vi "swerve_open_module.vi"(0 "Module Suffix":string, 5 "Drive CAN ID":u8, 7 "Azimuth CAN ID":u8, 9 "Encoder CAN ID":u8, 11 "error in":errorcluster, 12 "Encoder Offset (Deg)":dbl) -> (15 "error out":errorcluster)   [LabVIEW 2020]
uses:
  <vilib>/Rock Robotics/WPI/ThirdParty/Phoenix-LabVIEW/CANCoder/Controls/CTRE_Phoenix_CANcoder_AbsoluteSensorRange.ctl
  <vilib>/Rock Robotics/WPI/ThirdParty/Phoenix-LabVIEW/CANCoder/Controls/CTRE_Phoenix_CANcoder_StatusFrame.ctl
  <vilib>/Rock Robotics/WPI/ThirdParty/Phoenix-LabVIEW/Motor Controller/Controls/CTRE_Phoenix_MotorControl_FeedbackDevice_TalonFX.ctl
  <vilib>/Rock Robotics/WPI/ThirdParty/Phoenix-LabVIEW/Motor Controller/Controls/CTRE_Phoenix_MotorControl_RemoteSourceType.ctl
  <vilib>/Rock Robotics/WPI/ThirdParty/Phoenix-LabVIEW/Motor Controller/Controls/CTRE_Phoenix_MotorControl_NeutralMode.ctl
  <vilib>/Rock Robotics/WPI/ThirdParty/Phoenix-LabVIEW/CANCoder/Controls/CTRE_Phoenix_CANcoder_SensorInitializationStrategy.ctl
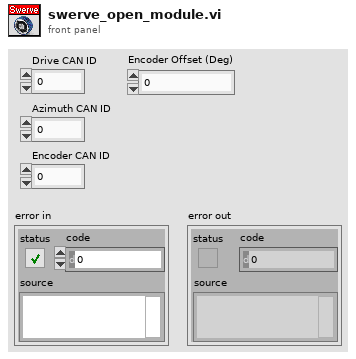
[diagram p1: front panel]
types:
  T1 = typedef "CTRE_Phoenix_CANcoder_StatusFrame.ctl" = u32
  T2 = typedef "CTRE_Phoenix_CANcoder_AbsoluteSensorRange.ctl" = enum16{"Unsigned [0 to 360)", "Signed [-180 to +180)"}
  T3 = typedef "CTRE_Phoenix_MotorControl_NeutralMode.ctl" = enum8{"EEPROMSetting", "Override to Coast", "Override to Brake"}
  T4 = typedef "CTRE_Phoenix_MotorControl_FeedbackDevice_TalonFX.ctl" = i8
  T5 = typedef "CTRE_Phoenix_MotorControl_RemoteSourceType.ctl" = enum16{"Off", "Talon SRX Selected Sensor", "Pigeon IMU Yaw", "Pigeon IMU Pitch", "Pigeon IMU Roll", "CANifier Quadrature", "CANifier PWM Input 0", "CANifier PWM Input 1", "CANifier PWM Input 2", "CANifier PWM Input 3", "Gadgeteer Pigeon Yaw", "Gadgeteer Pigeon Pitch", "Gadgeteer Pigeon Roll", "CANCoder"}
  T6 = typedef "CTRE_Phoenix_CANcoder_SensorInitializationStrategy.ctl" = enum16{"Boot To Zero", "Boot To Absolute Position"}
  T7 = typedef "WPI_MotorControlDeviceRef.ctl" = cluster{"DeviceStatus":errorcluster, "Type":T8, "PWM":cluster{"PWM Channel":T9, "DeadBand":T10}, "CAN":cluster{"Device Number":u8, "SetOutput VI Ref":variant, "GetOutput VI Ref":variant, "Enable VI Ref":variant, "Disable VI Ref":variant, "Data":variant}, "Invert":bool, "DIO PWM":cluster{"PWM \"Enable\" Channel":T9, "DIOChannel":T11, "PWM Rate":dbl}}
  T8 = typedef "WPI_MotorControlType.ctl" = enum16{"PWM", "CAN", "DIO PWM"}
  T9 = typedef "FPGA_DIOPWMChannel.ctl" = enum8{"PWM 0", "PWM 1", "PWM 2", "PWM 3", "PWM 4", "PWM 5", "PWM 6", "PWM 7", "PWM 8", "PWM 9", "PWM MXP 0", "PWM MXP 1", "PWM MXP 2", "PWM MXP 3", "PWM MXP 4", "PWM MXP 5", "PWM MXP 6", "PWM MXP 7", "PWM MXP 8", "PWM MXP 9", "Invalid"}
  T10 = typedef "WPI_PWMDeadband.ctl" = cluster{"Name":string, "maxPositivePwm":i32, "minPositivePwm":i32, "centerPwm":i32, "maxNegativePwm":i32, "minNegativePwm":i32, "angularRange":u16}
  T11 = typedef "FPGA_DIOChannel.ctl" = enum8{"DIO 0", "DIO 1", "DIO 2", "DIO 3", "DIO 4", "DIO 5", "DIO 6", "DIO 7", "DIO 8", "DIO 9", "DIO MXP 0", "DIO MXP 1", "DIO MXP 2", "DIO MXP 3", "DIO MXP 4", "DIO MXP 5", "DIO MXP 6", "DIO MXP 7", "DIO MXP 8", "DIO MXP 9", "DIO MXP 10", "DIO MXP 11", "DIO MXP 12", "DIO MXP 13", "DIO MXP 14", "DIO MXP 15", "SPI Port CS1", "SPI Port CS2", "SPI Port CS3", "SPI Port MISO", "SPI Port MOSI", "Invalid"}
  T12 = typedef "CTRE_Phoenix_CANcoder_DeviceRef.ctl" = cluster{"DeviceStatus":errorcluster, "Device Number":u8, "Handle":u64, "UsageFrame":u32, "Library Path":path}
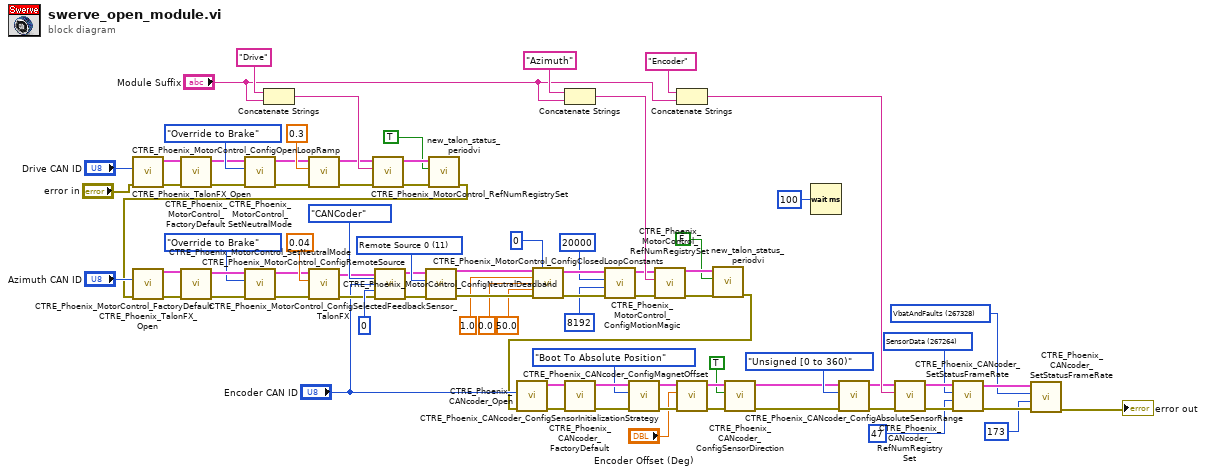
[diagram p0: block diagram]
diagram:
  w11 = T1 267328 items=["SensorData"=267264, "VbatAndFaults"=267328] ("CANcoder Status Frame")
  w21 = T1 267264 items=["SensorData"=267264, "VbatAndFaults"=267328] ("CANcoder Status Frame")
  w59 = T4 11 items=["Integrated Sensor"=1, "Sensor Sum (S0 + S1)"=9, "Sensor Difference (D0 - D1)"=10, "Remote Source 0"=11, "Remote Source 1"=12, "None"=14, "Software Emulated"=15] ("Talon FX Feedback Device")
  n1 = call <vilib>:"CTRE_Phoenix_TalonFX_Open.vi"("error in"="error in", "Device Number"="Drive CAN ID") -> ("error out"=w77:errorcluster, "PhoenixMotorControlDevRef"=w78:T7)  [unwired: 8 in]
  n2 = call <vilib>:"CTRE_Phoenix_MotorControl_FactoryDefault.vi"("error in"=w77, "PhoenixMotorControlDevRef"=w78) -> ("error out"=w30:errorcluster, "PhoenixMotorControlDevRef"=w31:T7)  [unwired: 8 in]
  n3 = call <vilib>:"CTRE_Phoenix_MotorControl_SetNeutralMode.vi"("error in (no error)"=w30, "Motor Control Neutral Mode"=CTRE_Phoenix_MotorControl_NeutralMode."Override to Brake", "PhoenixMotorControlDevRef"=w31) -> ("error out"=w28:errorcluster, "PhoenixMotorControlDevRef"=w29:T7)  [unwired: 7 in]
  n4 = Concatenate Strings("Drive" ("string"), "Module Suffix") -> (w79:string)
  n5 = call <vilib>:"CTRE_Phoenix_MotorControl_ConfigOpenLoopRamp.vi"("error in (no error)"=w28, "secondsFromNeutralToFull"=0.3 ("Drive Ramp (Sec)"), "PhoenixMotorControlDevRef"=w29) -> ("error out"=w26:errorcluster, "PhoenixMotorControlDevRef"=w27:T7)  [unwired: 7 in]
  n6 = call <vilib>:"CTRE_Phoenix_MotorControl_RefNumRegistrySet.vi"("error in (no error)"=w26, "refnum name"=w79, "PhoenixMotorControlDevRef"=w27) -> ("error out"=w4:errorcluster, "PhoenixMotorControlDevRef"=w3:T7)  [unwired: 7 in]
  n7 = call "new_talon_status_periodvi.vi"("error in (no error)"=w4, "Feedback Data?"=TRUE, "PhoenixMotorControlDevRef"=w3) -> ("error out"=w2:errorcluster)  [unwired: 7 in, 1 out]
  n8 = call <vilib>:"CTRE_Phoenix_TalonFX_Open.vi"("error in"=w2, "Device Number"="Azimuth CAN ID") -> ("error out"=w76:errorcluster, "PhoenixMotorControlDevRef"=w75:T7)  [unwired: 8 in]
  n9 = call <vilib>:"CTRE_Phoenix_MotorControl_FactoryDefault.vi"("error in"=w76, "PhoenixMotorControlDevRef"=w75) -> ("error out"=w49:errorcluster, "PhoenixMotorControlDevRef"=w50:T7)  [unwired: 8 in]
  n10 = call <vilib>:"CTRE_Phoenix_MotorControl_SetNeutralMode.vi"("error in (no error)"=w49, "Motor Control Neutral Mode"=CTRE_Phoenix_MotorControl_NeutralMode."Override to Brake", "PhoenixMotorControlDevRef"=w50) -> ("error out"=w47:errorcluster, "PhoenixMotorControlDevRef"=w48:T7)  [unwired: 7 in]
  n11 = call <vilib>:"CTRE_Phoenix_MotorControl_ConfigNeutralDeadband.vi"("error in (no error)"=w47, "Percent Deadband"=0.04, "PhoenixMotorControlDevRef"=w48) -> ("error out"=w44:errorcluster, "PhoenixMotorControlDevRef"=w45:T7)  [unwired: 7 in]
  n12 = call <vilib>:"CTRE_Phoenix_MotorControl_ConfigRemoteSource.vi"("PhoenixMotorControlDevRef"=w45, "Remote Device Type"=CTRE_Phoenix_MotorControl_RemoteSourceType."CANCoder", "Remote Device ID"="Encoder CAN ID", "Source Index (0/1)"=u32 0, "error in (no error)"=w44) -> ("PhoenixMotorControlDevRef"=w56:T7, "error out"=w55:errorcluster)  [unwired: 9 in]
  n13 = call <vilib>:"CTRE_Phoenix_MotorControl_ConfigSelectedFeedbackSensor_TalonFX.vi"("error in (no error)"=w55, "Talon FX Feedback Device"=w59, "PhoenixMotorControlDevRef"=w56) -> ("error out"=w42:errorcluster, "PhoenixMotorControlDevRef"=w43:T7)  [unwired: 7 in]
  n14 = call <vilib>:"CTRE_Phoenix_MotorControl_ConfigClosedLoopConstants.vi"("PhoenixMotorControlDevRef"=w43, "slotIdx"=0, "P"=1.0, "I"=0.0 ("P"), "D"=50.0 ("P"), "error in (no error)"=w42) -> ("PhoenixMotorControlDevRef"=w37:T7, "error out"=w36:errorcluster)  [unwired: 8 in]
  n15 = Concatenate Strings("Azimuth" ("string"), "Module Suffix") -> (w72:string)
  n16 = call <vilib>:"CTRE_Phoenix_MotorControl_ConfigMotionMagic.vi"("error in (no error)"=w36, "Acceleration"=8192 ("Cruise Velocity"), "Cruise Velocity"=20000, "PhoenixMotorControlDevRef"=w37) -> ("error out"=w32:errorcluster, "PhoenixMotorControlDevRef"=w33:T7)  [unwired: 6 in]
  n17 = call <vilib>:"CTRE_Phoenix_MotorControl_RefNumRegistrySet.vi"("error in (no error)"=w32, "refnum name"=w72, "PhoenixMotorControlDevRef"=w33) -> ("error out"=w7:errorcluster, "PhoenixMotorControlDevRef"=w8:T7)  [unwired: 7 in]
  n18 = Concatenate Strings("Encoder" ("string"), "Module Suffix") -> (w70:string)
  n19 = call "new_talon_status_periodvi.vi"("error in (no error)"=w7, "Feedback Data?"=FALSE, "PhoenixMotorControlDevRef"=w8) -> ("error out"=w6:errorcluster)  [unwired: 7 in, 1 out]
  n20 = call <vilib>:"CTRE_Phoenix_CANcoder_Open.vi"("error in"=w6, "Device Number"="Encoder CAN ID") -> ("error out"=w52:errorcluster, "CTRE_CANcoder_DeviceRef"=w53:T12)  [unwired: 8 in]
  n21 = call <vilib>:"CTRE_Phoenix_CANcoder_FactoryDefault.vi"("error in"=w52, "CTRE_CANcoder_DeviceRef"=w53) -> ("error out"=w69:errorcluster, "CTRE_CANcoder_DeviceRef"=w68:T12)  [unwired: 8 in]
  n22 = call <vilib>:"CTRE_Phoenix_CANcoder_ConfigSensorInitializationStrategy.vi"("error in"=w69, "Sensor Initialization Strategy"=CTRE_Phoenix_CANcoder_SensorInitializationStrategy."Boot To Absolute Position", "CTRE_CANcoder_DeviceRef"=w68) -> ("error out"=w65:errorcluster, "CTRE_CANcoder_DeviceRef"=w64:T12)  [unwired: 7 in]
  n23 = call <vilib>:"CTRE_Phoenix_CANcoder_ConfigMagnetOffset.vi"("error in"=w65, "Magnet Offset (Degrees)"="Encoder Offset (Deg)", "CTRE_CANcoder_DeviceRef"=w64) -> ("error out"=w62:errorcluster, "CTRE_CANcoder_DeviceRef"=w61:T12)  [unwired: 7 in]
  n24 = call <vilib>:"CTRE_Phoenix_CANcoder_ConfigSensorDirection.vi"("error in"=w62, "Sensor Direction"=TRUE, "CTRE_CANcoder_DeviceRef"=w61) -> ("error out"=w15:errorcluster, "CTRE_CANcoder_DeviceRef"=w16:T12)  [unwired: 7 in]
  n25 = Wait (ms)(milliseconds to wait=u32 100) -> ()  [unwired: 1 out]
  n26 = call <vilib>:"CTRE_Phoenix_CANcoder_ConfigAbsoluteSensorRange.vi"("error in"=w15, "Absolute Sensor Range"=CTRE_Phoenix_CANcoder_AbsoluteSensorRange."Unsigned [0 to 360)", "CTRE_CANcoder_DeviceRef"=w16) -> ("error out"=w19:errorcluster, "CTRE_CANcoder_DeviceRef"=w18:T12)  [unwired: 7 in]
  n27 = call <vilib>:"CTRE_Phoenix_CANcoder_RefNumRegistrySet.vi"("error in (no error)"=w19, "refnum name"=w70, "CTRE_CANcoder_DeviceRef"=w18) -> ("error out"=w23:errorcluster, "CTRE_CANcoder_DeviceRef"=w22:T12)  [unwired: 7 in]
  n28 = call <vilib>:"CTRE_Phoenix_CANcoder_SetStatusFrameRate.vi"("error in (no error)"=w23, "Period (ms)"=u8 47, "CANcoder Status Frame"=w21, "CTRE_CANcoder_DeviceRef"=w22) -> ("error out"=w12:errorcluster, "CTRE_CANcoder_DeviceRef"=w13:T12)  [unwired: 6 in]
  n29 = call <vilib>:"CTRE_Phoenix_CANcoder_SetStatusFrameRate.vi"("error in (no error)"=w12, "Period (ms)"=u8 173, "CANcoder Status Frame"=w11, "CTRE_CANcoder_DeviceRef"=w13) -> ("error out"=→"error out":errorcluster)  [unwired: 6 in, 1 out]
